vi "Buffer.vi"(5 "Parameters":T4={"Index"=0, "Size"=3000, "Samples"=0, "Ordered ?"=FALSE}, 7 "Mode":T2, 8 "Error IN":errorcluster, 10 "DATA IN":T1[](array[typedef])) -> (0 "Error OUT":errorcluster, 1 "Output":T3, 2 "DATA OUT":T1[](array[typedef]), 3 "New Element ?":bool, 4 "Index":i32)   [LabVIEW 2017, in "PMU data buffer.lvlib"]
uses:
  PMU data buffer.lvlib
  Buffer Settings.ctl
  Buffer DATA OUT ordered.ctl
  Buffer state.ctl
  Buffer DATA cluster.ctl
panel:
  # "Buffer Paremeters"
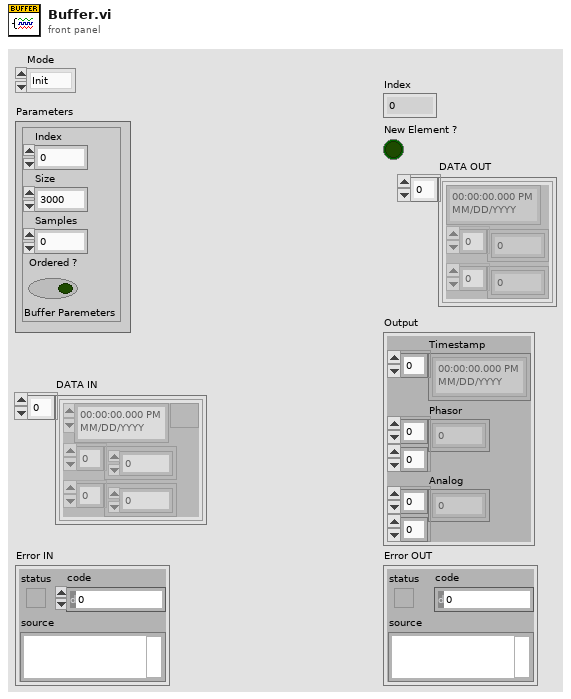
[diagram p1: front panel]
types:
  T1 = typedef "PMU data buffer.lvlib/Buffer DATA cluster.ctl" = cluster{timestamp, csg[], sgl[]}
  T2 = typedef "PMU data buffer.lvlib/Buffer state.ctl" = enum16{"Init", "Change Size", "Flush", "Exit", "Add", "Get", "Hist_Toggle", "Add_Serv"}
  T3 = typedef "PMU data buffer.lvlib/Buffer DATA OUT ordered.ctl" = cluster{"Timestamp":timestamp[], "Phasor":csg[][], "Analog":sgl[][]}
  T4 = typedef "PMU data buffer.lvlib/Buffer Settings.ctl" = cluster{"Index":i32, "Size":i32, "Samples":i32, "Ordered ?":bool}
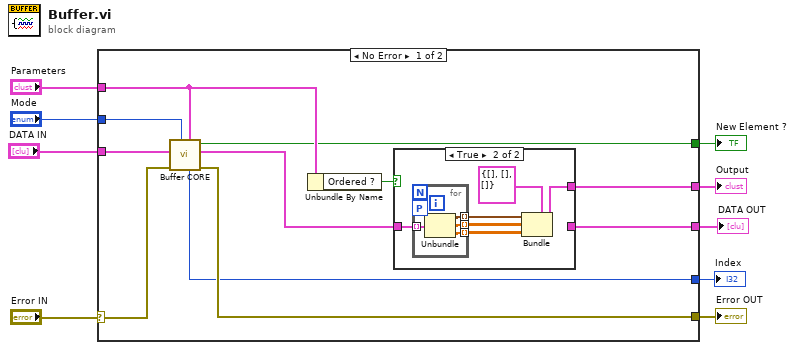
[diagram p0: block diagram]
diagram:
  n1 = case shown="No Error" "Error IN" {
    selector: "Error IN" -> [w18 w32]
    tunnel: "Mode" -> [w11 _]
    tunnel: [w17 w32] -> w9
    tunnel: "DATA IN" -> [w14 _]
    tunnel: [w19 _] -> w7
    tunnel: "Parameters" -> [w16 _]
    tunnel: [w13 _] -> w4
    tunnel: [w20 _] -> w1
    tunnel: [w12 _] -> w3
    frame No Error {
      n2 = call "Buffer CORE.vi"("Parameters"=w16, "Mode"=w11, "Error IN"=w18, "DATA IN"=w14) -> ("Error OUT"=w17:errorcluster, "DATA OUT"=w10:T1[], "New Element ?"=w13:bool, "Index"=w12:i32)  [unwired: 4 in]
      n3 = Unbundle By Name(w16) -> ("Ordered ?"=w15:bool)
      n4 = case shown="True" w15 {
        tunnel: w10 -> [w21 w23]
        tunnel: [w21 _] -> w20
        tunnel: [_ w24] -> w19
        frame False {
        }
        frame True {
          n5 = for {
            tunnel: w23 -> [w28] mode=indexing
            tunnel: [w31] -> w25 mode=indexing
            tunnel: [w30] -> w26 mode=indexing
            tunnel: [w29] -> w27 mode=indexing
            workers-P: _ -> [_]
            n6 = Unbundle(w28) -> (w31:timestamp, w30:csg[], w29:sgl[])
          }
          n7 = Bundle(cluster=T3 {"Timestamp"=[], "Phasor"=[], "Analog"=[]} ("Output"), "Timestamp"=w25, "Phasor"=w26, "Analog"=w27) -> (w24:T3)
        }
      }
    }
    frame Error {
    }
  }
  "Error OUT" <- w9
  "Output" <- w7
  "New Element ?" <- w4
  "Index" <- w3
  "DATA OUT" <- w1
